vi "ReceiveMessage.vi"(0 "STOMP in":refnum<class "STOMP.lvclass">, 3 "timeout ms (25000)":i32=25000, 5 "error in (no error)":errorcluster) -> (14 "STOMP out":refnum<class "STOMP.lvclass">, 16 "ServerFrame":T1, 19 "error out":errorcluster)   [LabVIEW 2017, in "LabVIEW STOMP.lvlib" / "STOMP.lvclass"]
uses:
  STOMP.lvclass
  Typedefs/Type_ServerFrame.ctl
  Typedefs/Type_ServerFrameType.ctl
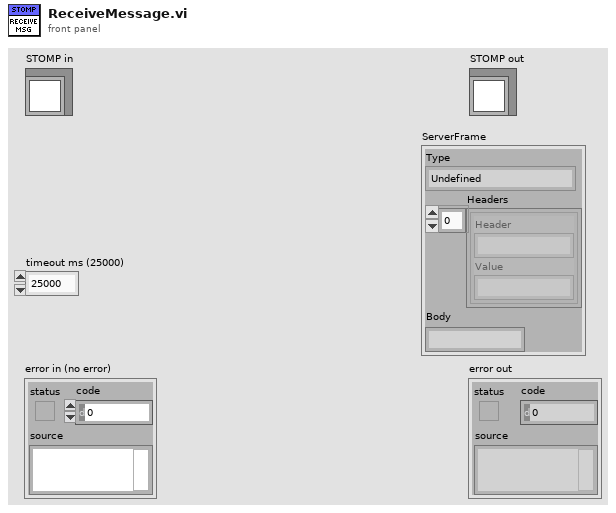
[diagram p1: front panel]
types:
  T1 = typedef "LabVIEW STOMP.lvlib/STOMP.lvclass/Type_ServerFrame.ctl" = cluster{"Type":T2, "Headers":cluster{"Header":string, "Value":string}[], "Body":string}
  T2 = typedef "LabVIEW STOMP.lvlib/STOMP.lvclass/Type_ServerFrameType.ctl" = enum16{"Undefined", "MESSAGE", "CONNECTED", "RECEIPT", "ERROR"}
  T3 = typedef "STOMP Connection Manager.lvclass/ObjectAttributes.ctl" = cluster{"address":string, "port":u16, "ConnectionRef":refnum<k5>, "messageQueue":refnum<queue>, "receiptQueue":refnum<queue>, "errorQueue":refnum<queue>, "sendQueue":refnum<queue>, "currentReceiptNumber":u64, "currentSubscriptionId":u64, "closeConnection":bool, "activeSubscriptions":T4[]}
  T4 = typedef "LabVIEW STOMP.lvlib/STOMP.lvclass/Type_ActiveSubscription.ctl" = cluster{"id":u64, "receipt":bool, "Destination":string, "ack":T5, "headers":T6[]}
  T5 = typedef "LabVIEW STOMP.lvlib/STOMP.lvclass/Type_AckHeader.ctl" = enum16{"auto", "client", "client-individual"}
  T6 = typedef "LabVIEW STOMP.lvlib/STOMP.lvclass/Type_FrameHeader.ctl" = cluster{"Header":string, "Value":string}
  T7 = enum16{"Standard", "Buffered", "CRLF", "Immediate"}
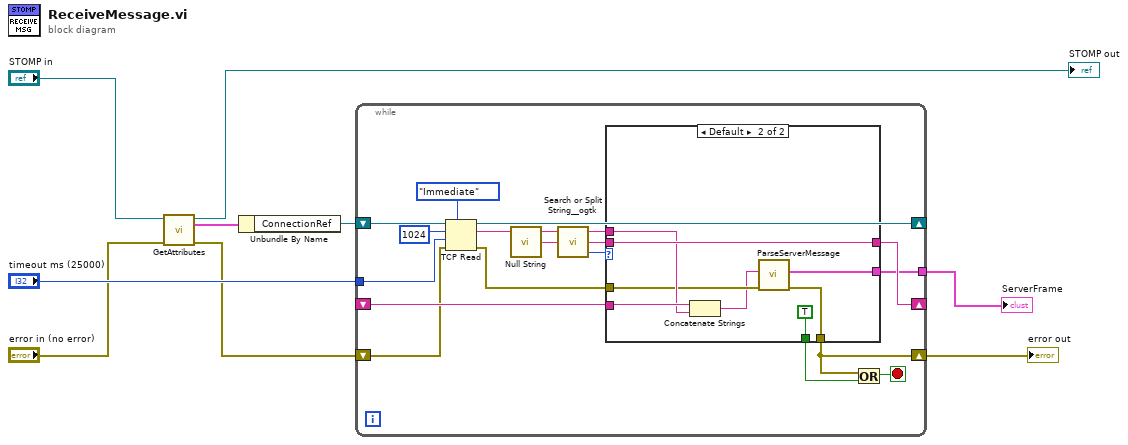
[diagram p0: block diagram]
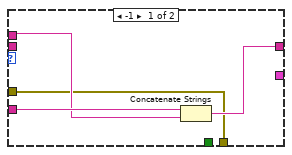
[diagram p2: hidden frame]
diagram:
  n1 = call-dynamic "GetAttributes.vi"("error in (no error)"="error in (no error)", "STOMP in"="STOMP in") -> ("error out"=w2:errorcluster, "attributes"=w4:T3, "STOMP out"=→"STOMP out":refnum<class "STOMP.lvclass">)  [unwired: 7 in]
  n2 = Unbundle By Name(w4) -> ("ConnectionRef"=w8:refnum<k5>)
  n3 = while {
    shift-right: [w24] -> _
    shift-left: w8 -> [w25]
    shift-right: [w15] -> _
    shift-left: _ -> [w22]
    shift-right: [w12] -> w6
    shift-left: w2 -> [w20]
    tunnel: "timeout ms (25000)" -> [w11]
    tunnel: [w10] -> w7
    stop <- w13 stop-if-true
    n4 = TCP Read(connection ID=w25, bytes to read=1024, error in (no error)=w20, 7:T7."Immediate" ("mode (standard)"), 9:w11) -> (connection ID out=w24:refnum<k5>, data out=w23:string, error out=w21:errorcluster)
    n5 = call "Null String.vi"() -> ("NULL"=w19:string)  [unwired: 19 in]
    n6 = call <userlib>:"Search or Split String__ogtk.vi"("search string/char (-)"=w19, "string"=w23) -> ("offset after match"=w17:i32, "substring after match"=w16:string, "substring before match"=w18:string)  [unwired: 1 in]
    n7 = case shown="Default" w17 {
      tunnel: w22 -> [w31 w39]
      tunnel: w21 -> [w28 w36]
      tunnel: [w28 w34] -> w12
      tunnel: w18 -> [w30 w37]
      tunnel: w16 -> [_ w38]
      tunnel: [w29 w38] -> w15
      tunnel: [_ TRUE] -> w14
      tunnel: [_ w32] -> w10
      frame -1 {
        n8 = Concatenate Strings(w31, w30) -> (w29:string)
      }
      frame Default {
        n9 = Concatenate Strings(w39, w37) -> (w35:string)
        n10 = call "ParseServerMessage.vi"("error in (no error)"=w36, "msg"=w35) -> ("error out"=w34:errorcluster, "ServerFrame"=w32:T1)  [unwired: 8 in]
      }
    }
    n11 = Or(x=w12, y=w14) -> (x .or. y?=w13:bool)
  }
  "error out" <- w6
  "ServerFrame" <- w7
